vi "EnQcmds.vi"(6 "timeout in ms (-1)":i32, 7 "priority?":bool, 8 "error in (no error)":errorcluster, 10 "commands":T2[](array[typedef]), 11 "EnQin":T1) -> (0 "error out":errorcluster, 3 "EnQout":T1, 4 "timed out?":bool)   [LabVIEW 2021]
uses:
  EnQcmd.ctl
  EnQref.ctl
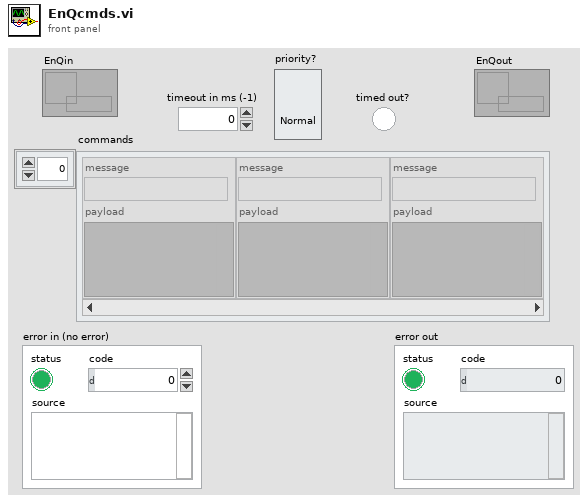
[diagram p1: front panel]
types:
  T1 = typedef "EnQref.ctl" = refnum<queue>
  T2 = typedef "EnQcmd.ctl" = cluster{"message":string, "payload":variant}
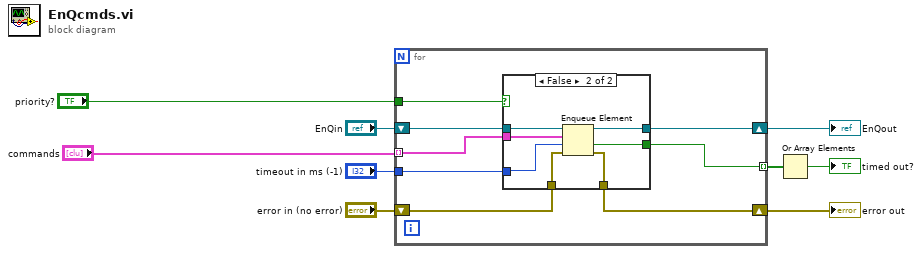
[diagram p0: block diagram]
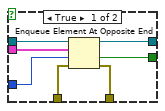
[diagram p2: hidden frame]
diagram:
  n1 = for {
    tunnel: [w13] -> w6 mode=indexing
    shift-right: [w16] -> w9
    shift-left: "EnQin" -> [w17]
    shift-right: [w14] -> w7
    shift-left: "error in (no error)" -> [w15]
    tunnel: "commands" -> [w12] mode=indexing
    tunnel: "priority?" -> [w11]
    tunnel: "timeout in ms (-1)" -> [w10]
    n2 = case shown="False" w11 {
      tunnel: w17 -> [w24 w31]
      tunnel: [w23 w30] -> w16
      tunnel: w15 -> [w22 w29]
      tunnel: [w21 w28] -> w14
      tunnel: [w20 w27] -> w13
      tunnel: w12 -> [w19 w26]
      tunnel: w10 -> [w18 w25]
      frame True {
        n3 = Enqueue Element At Opposite End(queue=w24, element=w19, timeout in ms (-1)=w18, error in (no error)=w22) -> (queue out=w23:T1, timed out?=w20:bool, error out=w21:errorcluster)
      }
      frame False {
        n4 = Enqueue Element(queue=w31, element=w26, timeout in ms (-1)=w25, error in (no error)=w29) -> (queue out=w30:T1, timed out?=w27:bool, error out=w28:errorcluster)
      }
    }
  }
  "error out" <- w7
  "EnQout" <- w9
  n5 = Or Array Elements(Boolean array=w6) -> (logical OR=→"timed out?":bool)
